vi "Read Orientation.vi"(8 "error in (no error)":errorcluster, 11 "Splitter in":refnum<class "Splitter.lvclass">) -> (0 "error out":errorcluster, 2 "Splitter Orientation":T1, 3 "Splitter out":refnum<class "Splitter.lvclass">)   [LabVIEW 2019, in "Splitter.lvclass"]
uses:
  <resource>/dialog/QuickDrop/plugins/PaneRelief/Classes/Splitter/Splitter.lvclass
  <resource>/dialog/QuickDrop/plugins/PaneRelief/Typedefs/Splitter Orientation--Enum.ctl
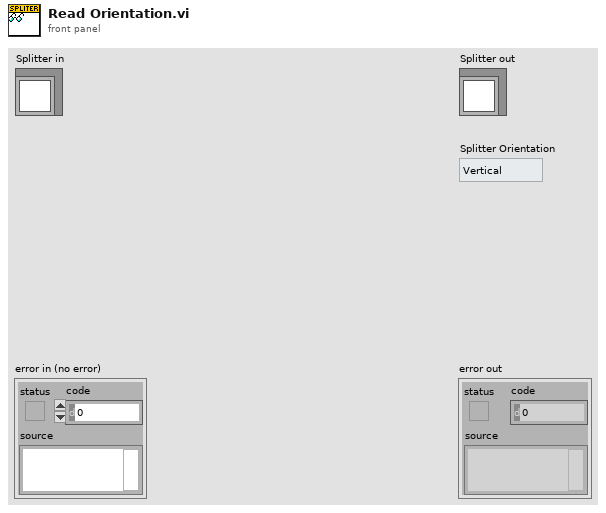
[diagram p1: front panel]
types:
  T1 = typedef "Splitter Orientation--Enum.ctl" = enum16{"Vertical", "Horizontal"}
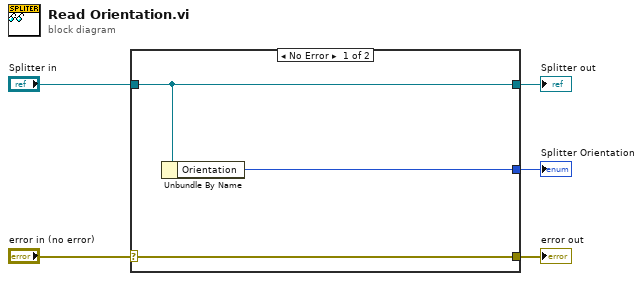
[diagram p0: block diagram]
diagram:
  n1 = case shown="No Error" "error in (no error)" {
    selector: "error in (no error)" -> [w8 w9]
    tunnel: [w8 w9] -> w4
    tunnel: [w7 w10] -> w2
    tunnel: "Splitter in" -> [w7 w10]
    tunnel: [w6 _] -> w1
    frame No Error {
      n2 = Unbundle By Name(w7) -> ("Orientation"=w6:T1)
    }
    frame Error {
    }
  }
  "error out" <- w4
  "Splitter out" <- w2
  "Splitter Orientation" <- w1
